vi "Startup.vi"() -> ()   [LabVIEW 2014]
uses:
  CustomControls/Program_States.ctl
  CustomControls/TSE_Status.ctl
  SharedVariables/TSE_Variables.vi
panel:
  out "String":string
  out "error out":errorcluster
  out "Status":string
  out "Ring":T1=enum."Ön Yükleme Tamam"
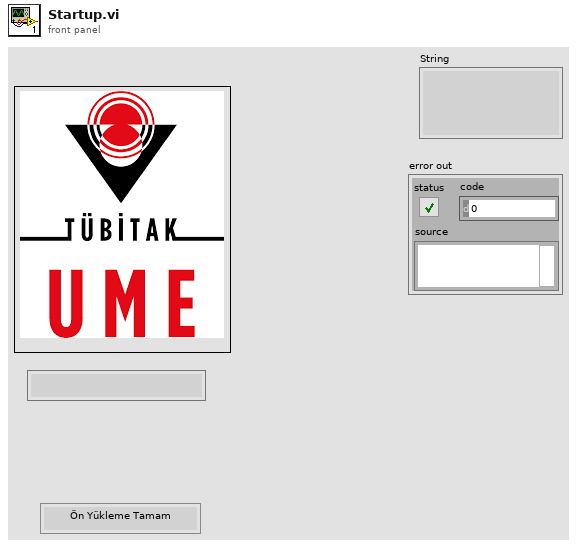
[diagram p1: front panel]
types:
  T1 = typedef "Program_States.ctl" = enum16{"Ön Yükleme", "TSE Baslat", "Kalibratöre Baglan", "Kalibratörü Baslat", "Ön Yükleme Tamam", "Frekans Testi", "Gerilim Testi", "Akim Testi", "Aktif Guc Testi", "Reaktif Guc Testi", "AC Akim Harmonik Testi", "AC Gerilim Harmonik Testi", "Flicker Testi", "Rapor Cikarma", "Yeniden Başlat", "Bekleme", "Durdur"}
  T2 = typedef "TSE_Status.ctl" = cluster{"Return Code":i32, "Message":string, "error in (no error)":errorcluster, "Program State":T1, "Test A. Suresi":u32}
  T3 = enum32{"invalid app kind", "Development System", "Run Time System", "Student Edition", "Embedded LabVIEW", "Evaluation", "Custom"}
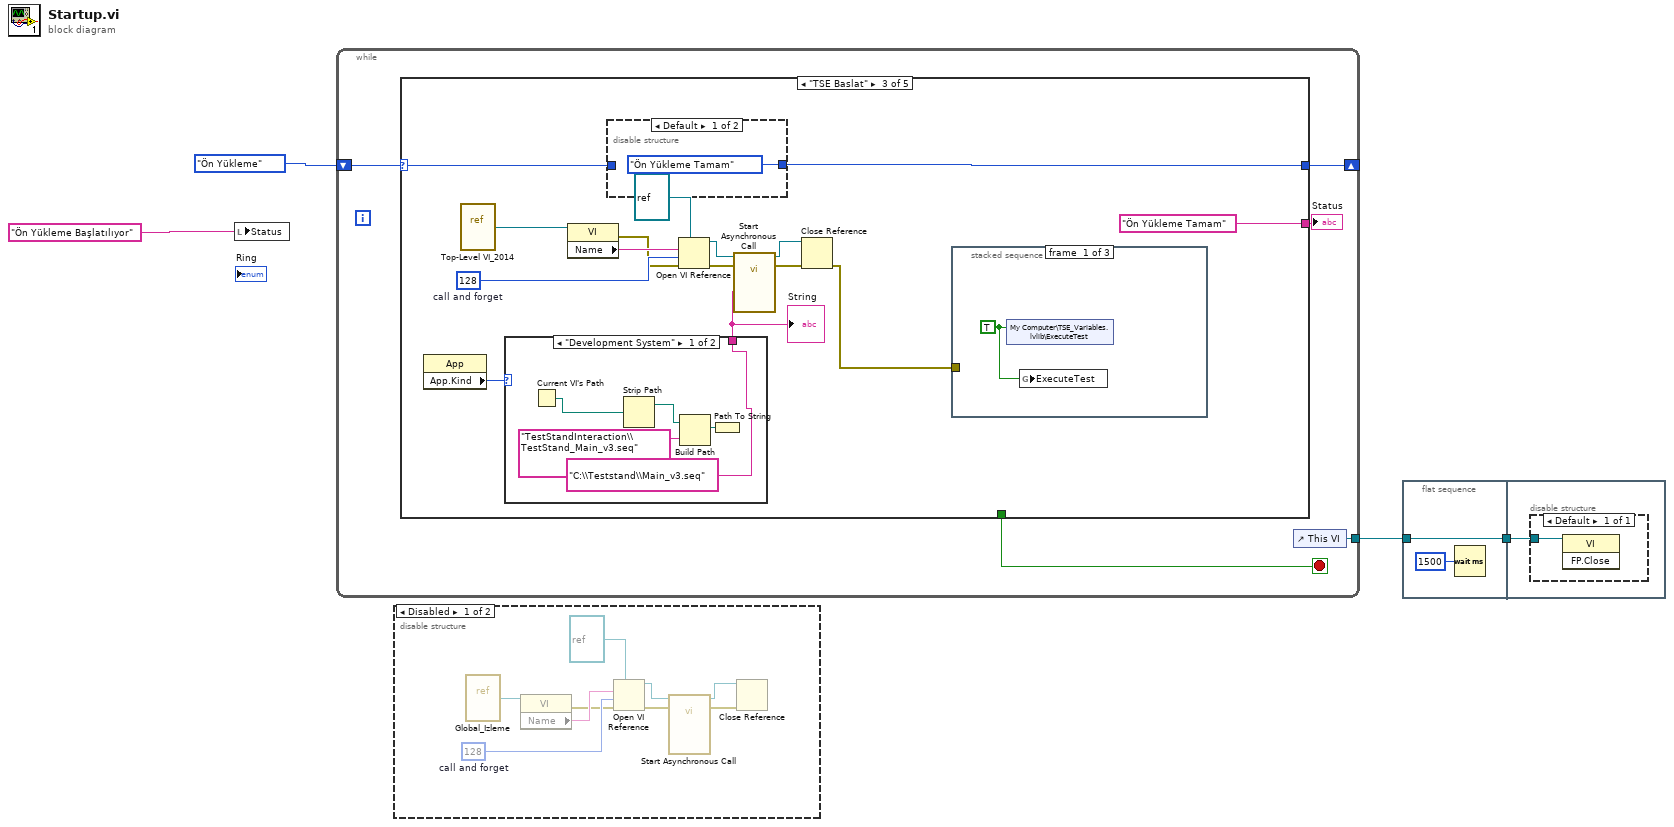
[diagram p0: block diagram]
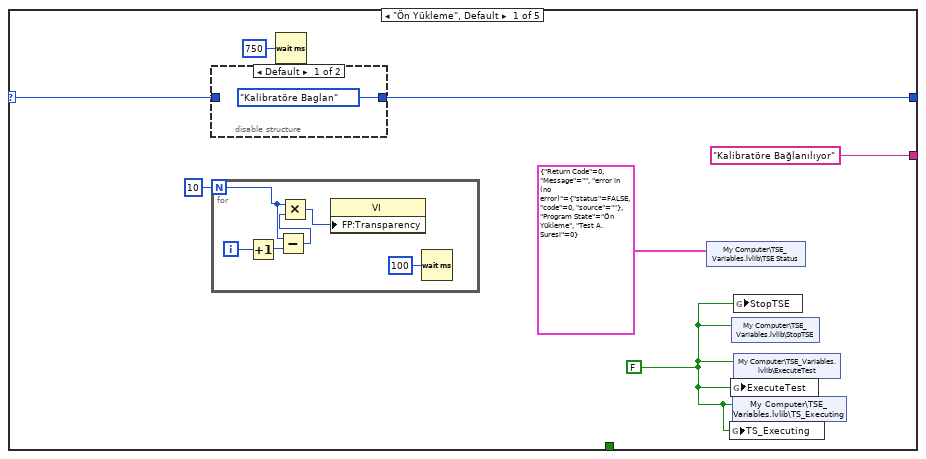
[diagram p3: hidden frame]
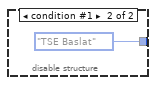
[diagram p4: hidden frame]
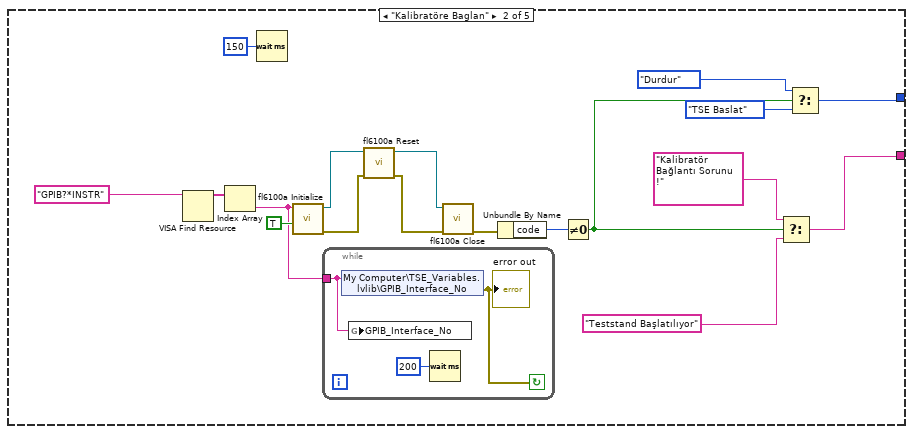
[diagram p5: hidden frame]
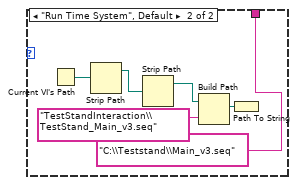
[diagram p6: hidden frame]
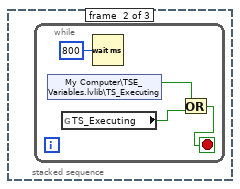
[diagram p7: hidden frame]
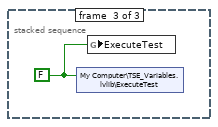
[diagram p8: hidden frame]
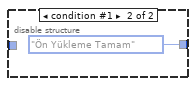
[diagram p9: hidden frame]
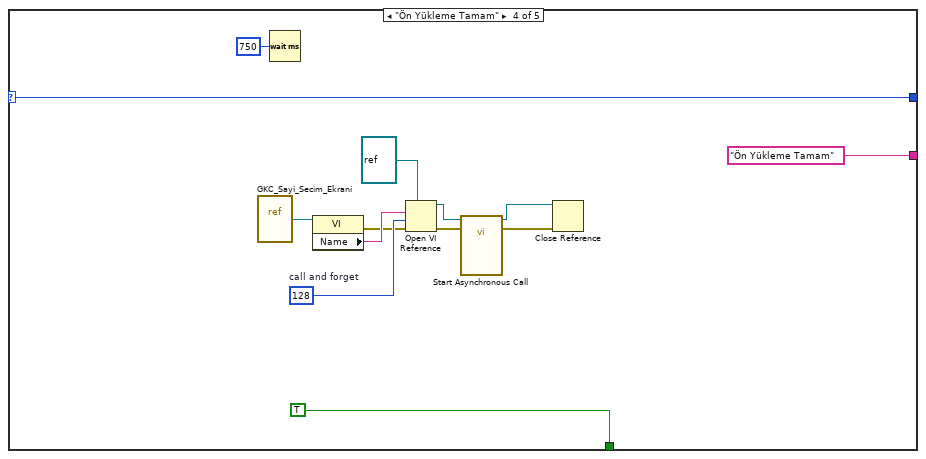
[diagram p10: hidden frame]
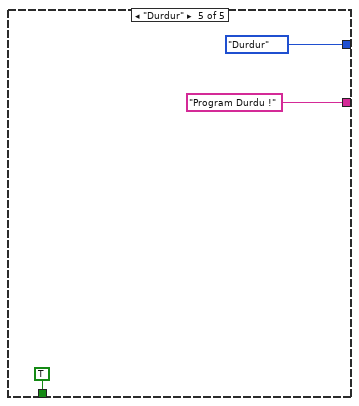
[diagram p11: hidden frame]
diagram:
  n1 = local write "Status"("Ön Yükleme Başlatılıyor" ("Status")) -> ()
  n2 = while {
    shift-right: [w9] -> _
    shift-left: Program_States."Ön Yükleme" ("Ring") -> [w6]
    tunnel: [w7] -> w3
    stop <- w8 stop-if-true
    n3 = case shown="\"TSE Baslat\"" w6 {
      selector: w6 -> [w16 _ w60 w81 _]
      tunnel: [w13 w33 w50 w81 Program_States."Durdur" ("Ring")] -> w9
      tunnel: [_ _ _ TRUE TRUE] -> w8
      tunnel: ["Kalibratöre Bağlanılıyor" ("f") w40 "Ön Yükleme Tamam" ("f") "Ön Yükleme Tamam" ("f") "Program Durdu !" ("f")] -> w5
      frame "Ön Yükleme", Default {
        w10 = FALSE ("ExecuteTest")
        n4 = disable-structure shown="Default" {
          disable-tunnel: [Program_States."Kalibratöre Baglan" Program_States."TSE Baslat"] -> w13
          disable-tunnel: w16 -> [_ _]
          frame condition #0 (active) {
          }
          frame condition #1 {
          }
        }
        n5 = for {
          N: 10 -> [w21]
          i -> [w24]
          n6 = Increment(x=w24) -> (x+1=w20:i32)
          n7 = Subtract(x=w21, y=w20) -> (x-y=w19:i32)
          n8 = Multiply(x=w21, y=w19) -> (x*y=w23:i32)
          n9 = property class="VI"("FP:Transparency"=w23) -> ()  [unwired: 2 in, 2 out]
          n10 = Wait (ms)(milliseconds to wait=u32 100) -> ()  [unwired: 1 out]
        }
        n11 = Wait (ms)(milliseconds to wait=u32 750) -> ()  [unwired: 1 out]
        n12 = shared-variable "My Computer\\TSE_Variables.lvlib\\TSE Status"(T2 {"Return Code"=0, "Message"="", "error in (no error)"={"status"=FALSE, "code"=0, "source"=""}, "Program State"=enum."Ön Yükleme", "Test A. Suresi"=0} ("TSE_Status_In")) -> ()  [unwired: 1 in, 1 out]
        n13 = global write "TSE_Variables.vi" "TS_Executing"(w10) -> ()
        n14 = global write "TSE_Variables.vi" "ExecuteTest"(w10) -> ()
        n15 = shared-variable "My Computer\\TSE_Variables.lvlib\\StopTSE"(w10) -> ()  [unwired: 1 in, 1 out]
        n16 = shared-variable "My Computer\\TSE_Variables.lvlib\\TS_Executing"(w10) -> ()  [unwired: 1 in, 1 out]
        n17 = global write "TSE_Variables.vi" "StopTSE"(w10) -> ()
        n18 = shared-variable "My Computer\\TSE_Variables.lvlib\\ExecuteTest"(w10) -> ()  [unwired: 1 in, 1 out]
      }
      frame "Kalibratöre Baglan" {
        n19 = VISA Find Resource(11:"GPIB?*INSTR" ("expression (\"?*\")")) -> (3:w37:string[])  [unwired: 2 in, 2 out]
        n20 = Index Array(array=w37) -> (element=w25:string)  [unwired: 1 in]
        n21 = Wait (ms)(milliseconds to wait=u32 150) -> ()  [unwired: 1 out]
        n22 = call <instrlib>:"fl6100a Initialize.vi"("Reset? (T: Yes)"=TRUE, "VISA resource name"=w25) -> ("error out"=w29:errorcluster, "VISA resource name out"=w30:refnum<visa-resource-name>)  [unwired: 8 in]
        n23 = while {
          tunnel: w25 -> [w45]
          stop <- w43 continue-if-true
          n24 = shared-variable "My Computer\\TSE_Variables.lvlib\\GPIB_Interface_No"(w45) -> (error out=w43:errorcluster)  [unwired: 1 in]
          "error out" <- w43
          n25 = global write "TSE_Variables.vi" "GPIB_Interface_No"(w45) -> ()
          n26 = Wait (ms)(milliseconds to wait=u32 200) -> ()  [unwired: 1 out]
        }
        n27 = call <instrlib>:"fl6100a Reset.vi"("error in (no error)"=w29, "VISA resource name"=w30) -> ("error out"=w28:errorcluster, "VISA resource name out"=w27:refnum<visa-resource-name>)  [unwired: 8 in]
        n28 = call <instrlib>:"fl6100a Close.vi"("error in (no error)"=w28, "VISA resource name"=w27) -> ("error out"=w35:errorcluster)  [unwired: 9 in]
        n29 = Unbundle By Name(w35) -> ("code"=w41:i32)
        n30 = Not Equal To 0?(x=w41) -> (x != 0?=w34:bool)
        n31 = Select(t="Kalibratör Bağlantı Sorunu !" ("f"), s=w34, f="Teststand Başlatılıyor") -> (s? t:f=w40:string)
        n32 = Select(t=Program_States."Durdur" ("Ring"), s=w34, f=Program_States."TSE Baslat") -> (s? t:f=w33:T1)
      }
      frame "TSE Baslat" {
        w59 = 128  # call and forget
        n33 = property class="App"() -> ("App.Kind"=w47:T3)  [unwired: 2 in, 2 out]
        n34 = vi-ref "Top-Level VI_2014.vi"() -> (w55:refnum<vi>)
        n35 = case shown="\"Development System\"" w47 {
          tunnel: ["C:\\Teststand\\Main_v3.seq" ("name or relative path") "C:\\Teststand\\Main_v3.seq" ("name or relative path")] -> w46
          frame "Development System" {
            n36 = Current VI's Path() -> (path=w62:path)
            n37 = Strip Path(path=w62) -> (stripped path=w65:path)  [unwired: 1 out]
            n38 = Build Path(base path=w65, name or relative path="TestStandInteraction\\TestStand_Main_v3.seq") -> (appended path=w63:path)
            n39 = Path To String(path=w63) -> ()  [unwired: 1 out]
          }
          frame "Run Time System", Default {
            n40 = Current VI's Path() -> (path=w71:path)
            n41 = Strip Path(path=w71) -> (stripped path=w70:path)  [unwired: 1 out]
            n42 = Strip Path(path=w70) -> (stripped path=w69:path)  [unwired: 1 out]
            n43 = Build Path(base path=w69, name or relative path="TestStandInteraction\\TestStand_Main_v3.seq") -> (appended path=w67:path)
            n44 = Path To String(path=w67) -> ()  [unwired: 1 out]
          }
        }
        "String" <- w46
        n45 = property class="VI"(reference=w55) -> (error out=w53:errorcluster, "Name"=w54:string)  [unwired: 1 in, 1 out]
        n46 = disable-structure shown="Default" {
          disable-tunnel: w60 -> [_ _]
          disable-tunnel: [Program_States."Ön Yükleme Tamam" Program_States."Ön Yükleme Tamam"] -> w50
          frame condition #0 (active) {
          }
          frame condition #1 {
          }
        }
        n47 = Open VI Reference(type specifier VI Refnum (for type only)=refnum<vi> refnum, vi path=w54, options=w59, error in (no error)=w53) -> (vi reference=w51:refnum<vi>, error out=w58:errorcluster)  [unwired: 2 in]
        n48 = call-by-ref "Start Asynchronous Call"(reference=w51, error in=w58, "sequenceFilePath"=w46) -> (reference out=w56:refnum<vi>, error out=w57:errorcluster)
        n49 = Close Reference(reference=w56, error in (no error)=w57) -> (error out=w49:errorcluster)
        n50 = stacked-sequence {
          tunnel: w49 -> [_ _ _]
          frame #0 {
            w72 = TRUE ("ExecuteTest")
            n51 = shared-variable "My Computer\\TSE_Variables.lvlib\\ExecuteTest"(w72) -> ()  [unwired: 1 in, 1 out]
            n52 = global write "TSE_Variables.vi" "ExecuteTest"(w72) -> ()
          }
          frame #1 {
            n53 = while {
              stop <- w74 stop-if-true
              n54 = shared-variable "My Computer\\TSE_Variables.lvlib\\TS_Executing"() -> (w75:bool)  [unwired: 1 in, 1 out]
              n55 = global read "TSE_Variables.vi" "TS_Executing"() -> (w73:bool)
              n56 = Wait (ms)(milliseconds to wait=u32 800) -> ()  [unwired: 1 out]
              n57 = Or(x=w75, y=w73) -> (x .or. y?=w74:bool)
            }
          }
          frame #2 {
            w77 = FALSE ("ExecuteTest")
            n58 = shared-variable "My Computer\\TSE_Variables.lvlib\\ExecuteTest"(w77) -> ()  [unwired: 1 in, 1 out]
            n59 = global write "TSE_Variables.vi" "ExecuteTest"(w77) -> ()
          }
        }
      }
      frame "Ön Yükleme Tamam" {
        w90 = 128  # call and forget
        n60 = vi-ref "GKC_Sayi_Secim_Ekrani.vi"() -> (w86:refnum<vi>)
        n61 = Wait (ms)(milliseconds to wait=u32 750) -> ()  [unwired: 1 out]
        n62 = property class="VI"(reference=w86) -> (error out=w84:errorcluster, "Name"=w85:string)  [unwired: 1 in, 1 out]
        n63 = Open VI Reference(type specifier VI Refnum (for type only)=refnum<vi> refnum, vi path=w85, options=w90, error in (no error)=w84) -> (vi reference=w82:refnum<vi>, error out=w89:errorcluster)  [unwired: 2 in]
        n64 = call-by-ref "Start Asynchronous Call"(reference=w82, error in=w89) -> (reference out=w87:refnum<vi>, error out=w88:errorcluster)  [unwired: 12 in]
        n65 = Close Reference(reference=w87, error in (no error)=w88) -> ()  [unwired: 1 out]
      }
      frame "Durdur" {
      }
    }
    "Status" <- w5
    n66 = control-ref of="This VI"() -> (w7:refnum<vi>)
  }
  n67 = disable-structure shown="Disabled" {
    frame Disabled {
      w104 = 128  # call and forget
      n68 = vi-ref "Global_Izleme.vi"() -> (w100:refnum<vi>)
      n69 = property class="VI"(reference=w100) -> (error out=w98:errorcluster, "Name"=w99:string)  [unwired: 1 in, 1 out]
      n70 = Open VI Reference(type specifier VI Refnum (for type only)=refnum<vi> refnum, vi path=w99, options=w104, error in (no error)=w98) -> (vi reference=w96:refnum<vi>, error out=w103:errorcluster)  [unwired: 2 in]
      n71 = call-by-ref "Start Asynchronous Call"(reference=w96, error in=w103) -> (reference out=w101:refnum<vi>, error out=w102:errorcluster)  [unwired: 12 in]
      n72 = Close Reference(reference=w101, error in (no error)=w102) -> ()  [unwired: 1 out]
    }
    frame Enabled {
    }
  }
  n73 = flat-sequence {
    tunnel: w3 -> [w106]
    tunnel: [w106] -> w2
    tunnel: w2 -> [w107]
    frame #0 {
      n74 = Wait (ms)(milliseconds to wait=u32 1500) -> ()  [unwired: 1 out]
    }
    frame #1 {
      n75 = disable-structure shown="Default" {
        disable-tunnel: w107 -> [w108]
        frame Enabled {
          n76 = invoke class="VI" method="FP.Close"(reference=w108) -> ()  [unwired: 2 in, 3 out]
        }
      }
    }
  }
